vi "Load New Launcher.vi"(6 "Loader Name Override":string, 8 "error in (no error)":errorcluster, 9 "Plugin Loader Path Override":path, 10 "Loader Load Info":T1, 11 "CIFPluginManager in":refnum<class "CIFPluginManager.lvclass">) -> (0 "error out":errorcluster)   [LabVIEW 2021, in "CIFPluginManager.lvclass"]
uses:
  CIFPluginManager.lvclass
  typedef/Loader Load Info.ctl
  typedef/Loader Type.ctl
  CIFPluginManager.lvclass/CIFPluginManager.ctl
  typedef/Loaders.ctl
  <vilib>/gRPC/LabVIEW gRPC Library/Shared/grpcId.ctl
  <vilib>/gRPC/LabVIEW gRPC Library/grpc-lvsupport-release.lvlib
  Engine Launch/CIF Engine Launch.lvlib
  <vilib>/CIF Foundation/CIF Utilities/Time/Time_CIF_U.lvlib
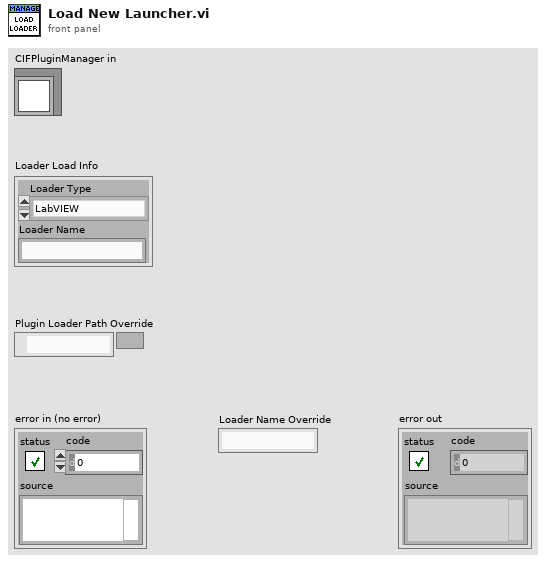
[diagram p1: front panel]
types:
  T1 = typedef "CIFPluginManager.lvclass/Loader Load Info.ctl" = cluster{"Loader Type":T2, "Loader Name":string}
  T2 = typedef "CIFPluginManager.lvclass/Loader Type.ctl" = enum16{"LabVIEW"}
  T3 = typedef "CIFPluginManager.lvclass/Loaders.ctl" = cluster{"Loader Type":T2, "grpc_port":i32, "pid":u32, "gRPC ID":T4, "Load Timestamp":i64, "Unloading":bool, "Ready for removal":bool, "Unload Timestamp":i64}
  T4 = typedef "grpc-lvsupport-release.lvlib/grpcId.ctl" = u64
  T5 = typedef "CIFPluginManager.lvclass/Loader Map.ctl" = map{string, T3}
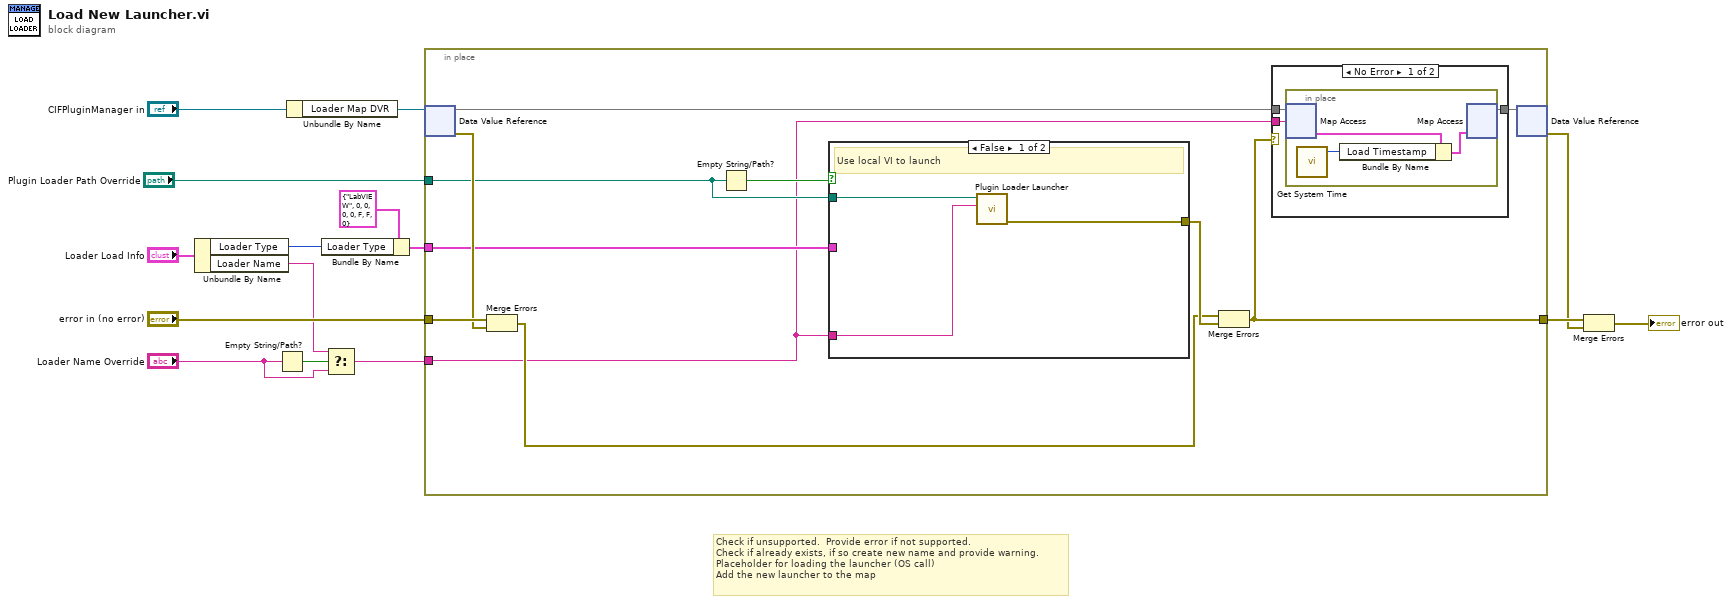
[diagram p0: block diagram]
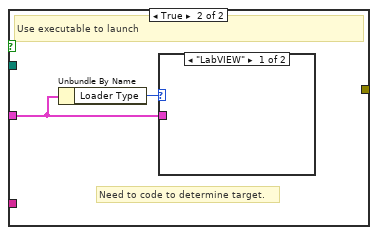
[diagram p3: hidden frame]
diagram:
  # "Check if unsupported.  Provide error if not supported.\nCheck if already exists, if so create new name and provide warning.\nPlaceholder for loading the launcher (OS call)\nAdd the new launcher to the map"
  n1 = Unbundle By Name("Loader Load Info") -> ("Loader Type"=w1:T2, "Loader Name"=w4:string)
  n2 = Empty String/Path?(string/path="Loader Name Override") -> (empty?=w6:bool)
  n3 = Unbundle By Name("CIFPluginManager in") -> ("Loader Map DVR"=w13:refnum<data-value>)
  n4 = Bundle By Name(cluster=T3 {"Loader Type"=enum."LabVIEW", "grpc_port"=0, "pid"=0, "gRPC ID"=0, "Load Timestamp"=0, "Unloading"=FALSE, "Ready for removal"=FALSE, "Unload Timestamp"=0} ("Launchers"), "Loader Type"=w1) -> (w9:T3)
  n5 = Select(t=w4, s=w6, f="Loader Name Override") -> (s? t:f=w3:string)
  n6 = in-place {
    in-place-border: "error in (no error)" -> [w26]
    in-place-border: [w16] -> w12
    in-place-border: w3 -> [w18]
    in-place-border: w9 -> [w23]
    in-place-border: "Plugin Loader Path Override" -> [w24]
    n7 = in-place-dvr #1(w13) -> (w19:T5, w25:errorcluster)
    n8 = Merge Errors(w26, w25) -> (w20:errorcluster)
    n9 = Empty String/Path?(string/path=w24) -> (empty?=w22:bool)
    n10 = case shown="False" w22 {
      tunnel: w24 -> [w36 _]
      tunnel: w23 -> [_ w37]
      tunnel: [w35 _] -> w21
      tunnel: w18 -> [w34 _]
      frame False {
        # "Use local VI to launch"
        n11 = call "Plugin Loader Launcher.vi"("Loader Name Override"=w34, "Plugin Loader Path Override"=w36) -> ("error out"=w35:errorcluster)  [unwired: 9 in]
      }
      frame True {
        # "Need to code to determine target."
        # "Use executable to launch"
        n12 = Unbundle By Name(w37) -> ("Loader Type"=w38:T2)
        n13 = case shown="\"LabVIEW\"" w38 {
          tunnel: w37 -> [_ _]
          frame "LabVIEW" {
          }
          frame Default {
          }
        }
      }
    }
    n14 = Merge Errors(w20, w21) -> (w16:errorcluster)
    n15 = case shown="No Error" w16 {
      tunnel: w19 -> [w29 w33]
      tunnel: w18 -> [w28 _]
      tunnel: [w27 w33] -> w17
      frame No Error {
        n16 = in-place {
          n17 = in-place-map #2(w29, w28) -> (w32:T3)  [unwired: 1 in, 1 out]
          n18 = call <vilib>:"Get System Time.vi"() -> ("Time (ns)"=w31:i64)  [unwired: 5 in]
          n19 = Bundle By Name(cluster=w32, "Load Timestamp"=w31) -> (w30:T3)
          n20 = in-place-map #2(w30) -> (w27:T5)  [unwired: 1 in, 2 out]
        }
      }
      frame Error {
      }
    }
    n21 = in-place-dvr #1(w17) -> (w11:errorcluster)  [unwired: 1 out]
  }
  n22 = Merge Errors(w12, w11) -> (→"error out":errorcluster)
